vi "Host Approach Retraction2(1)2.vi"() -> ()   [LabVIEW 2012]
uses:
  <vilib>/rvi/interface/nirviOpenFPGA/nirviOpenFPGA.xnode
  <vilib>/rvi/interface/nirviReadWriteControl/nirviReadWriteControl.xnode
  <vilib>/rvi/interface/nirviCloseFPGA/nirviCloseFPGA.xnode
  <vilib>/FPGAPlugInAG/Dynamic/niLvFpga_Close_Dynamic.vi
  <vilib>/rvi/interface/Simulation/niFpgaSimulationCallBeginRW.vi
  <vilib>/rvi/errors/niLvFpgaAdjustHostInterfaceError.vi
  <vilib>/rvi/interface/nirviMethod/nirviMethod.xnode
  <vilib>/FPGAPlugInAG/Dynamic/niLvFpga_Run_Dynamic.vi
  <vilib>/FPGAPlugInAG/PCI-7831R/niLvFpga_Open_PCI-7831R.vi
  <vilib>/rvi/interface/common/dynamic/niFpgaDynamicAddResources.vi
  <vilib>/Utility/error.llb/Error Cluster From Error Code.vi
  <vilib>/rvi/errors/niLvFpgaMergeErrorWithErrorCode.vi
  <vilib>/FPGAPlugInAG/Dynamic/niLvFpga_StartFifo_Dynamic.vi
  <vilib>/FPGAPlugInAG/Dynamic/niLvFpga_StopFifo_Dynamic.vi
  <vilib>/FPGAPlugInAG/Dynamic/niLvFpga_ReadFifo_Dynamic.vi
  SB130-XPS/Documents/FPGA-project-apporach-retraction/FPGA Bitfiles/Apporach-Retract_FPGATarget2_FPGATargetApproa_hZApBjrwAY4.lvbitx
  FPGA Target Approach Retraction2(1).vi
  NiFpgaLv.dll
panel:
  out "H/V  10":i16[](graph)
  out "Tuning Fork Signal":i16[](graph)
  out "Array":i64[](array[numeric])
  in  "Number of Elements":u16
  out "Counter Indicator":i32(graph)
  out "Z Indicator":dbl(graph)
  out "FPGA Output Voltage":dbl(graph)
  in  "MCL Counter":i64
  in  "MCL Divisions":i32
  out "MCL Range Indicator":bool
  out "Host Counter Indicator":i64
  out "Digital Steps per Region":i32
  out "Host Counter Output":i32
  in  "Z Position MCL Fine":i32
  out "Host Z Position Indicator":i32
  out "Z Position Range Indicator":bool
  out "Z Fine Steps per Region":dbl
  out "Host Z Output":fxp<+/-,40,30>
  in  "Manual Approach Start":bool
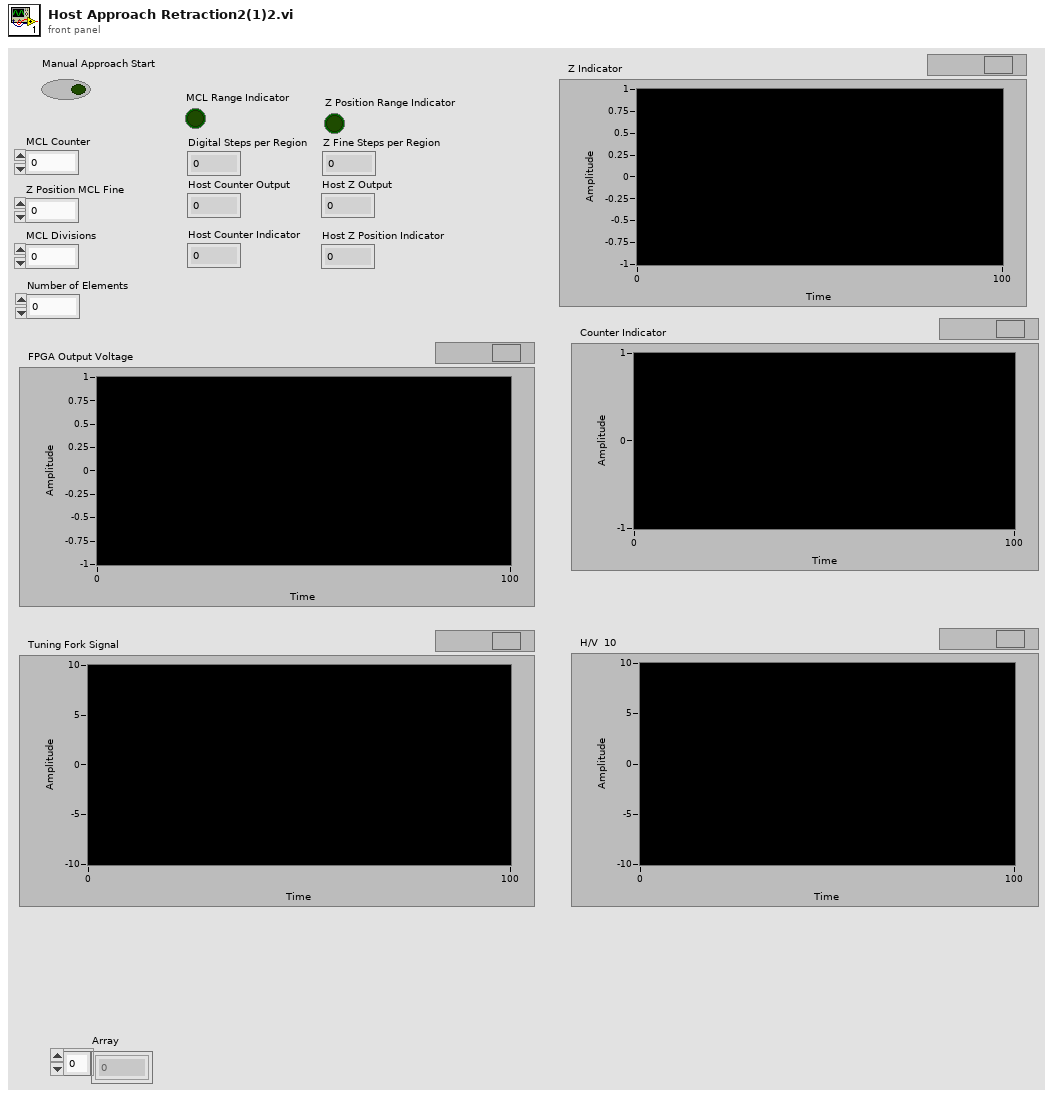
[diagram p1: front panel]
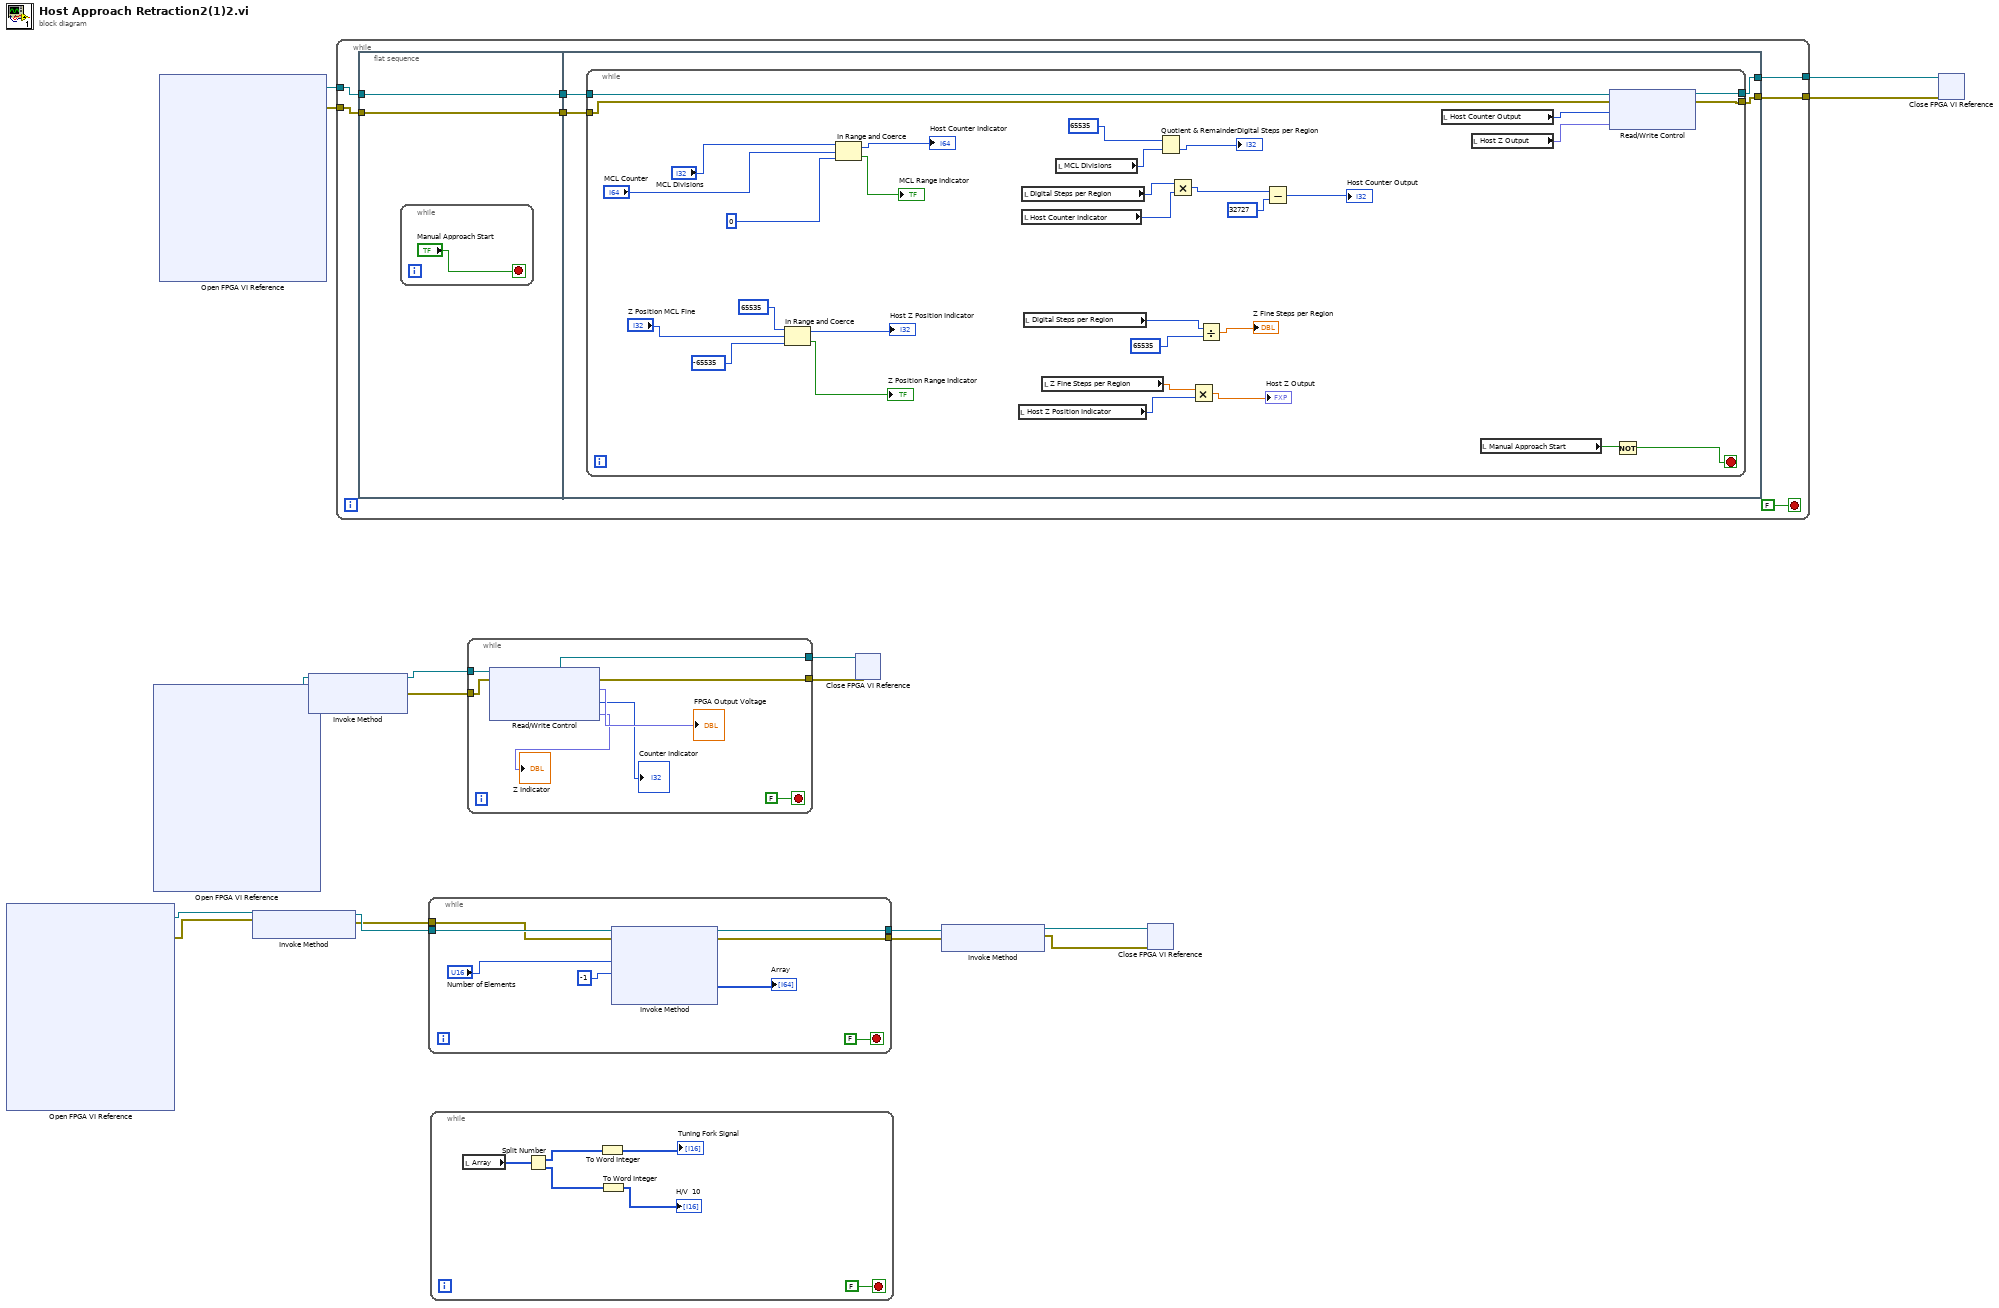
[diagram p0: block diagram]
diagram:
  n1 = xnode "Open FPGA VI Reference"() -> ("FPGA VI Reference Out"=w8:refnum<k20>, "error out"=w7:errorcluster)  [unwired: 2 in]
  n2 = xnode "Open FPGA VI Reference"() -> ("FPGA VI Reference Out"=w10:refnum<k20>, "error out"=w9:errorcluster)  [unwired: 2 in]
  n3 = xnode "Open FPGA VI Reference"() -> ("FPGA VI Reference Out"=w16:refnum<k20>, "error out"=w15:errorcluster)  [unwired: 2 in]
  n4 = xnode "Invoke Method"("FPGA VI Reference In"=w8, "error in"=w7) -> ("FPGA VI Reference Out"=w6:refnum<k20>, "error out"=w5:errorcluster)
  n5 = xnode "Invoke Method"("FPGA VI Reference In"=w10, "error in"=w9) -> ("FPGA VI Reference Out"=w12:refnum<k20>, "error out"=w11:errorcluster)  [unwired: 1 in]
  n6 = while {
    tunnel: [w24] -> w18
    tunnel: [w23] -> w17
    tunnel: w16 -> [w21]
    tunnel: w15 -> [w19]
    stop <- FALSE stop-if-true
    n7 = flat-sequence {
      tunnel: [w27] -> w22
      tunnel: w21 -> [w27]
      tunnel: [w26] -> w20
      tunnel: w19 -> [w26]
      tunnel: [w30] -> w24
      tunnel: [w29] -> w23
      tunnel: w22 -> [w32]
      tunnel: w20 -> [w31]
      frame #0 {
        n8 = while {
          stop <- "Manual Approach Start" stop-if-true
        }
      }
      frame #1 {
        n9 = while {
          tunnel: w32 -> [w64]
          tunnel: w31 -> [w63]
          tunnel: [w62] -> w30
          tunnel: [w61] -> w29
          stop <- w59 stop-if-true
          n10 = In Range and Coerce(upper limit=65535, x="Z Position MCL Fine", lower limit=-65535) -> (coerced(x)=→"Host Z Position Indicator":i32, In Range?=→"Z Position Range Indicator":bool)
          n11 = In Range and Coerce(upper limit="MCL Divisions", x="MCL Counter", lower limit=0) -> (coerced(x)=→"Host Counter Indicator":i64, In Range?=→"MCL Range Indicator":bool)
          n12 = local read "Host Z Position Indicator"() -> (w35:i32)
          n13 = local read "Digital Steps per Region"() -> (w48:i32)
          n14 = local read "Host Counter Indicator"() -> (w47:i64)
          n15 = local read "Digital Steps per Region"() -> (w39:i32)
          n16 = local read "Z Fine Steps per Region"() -> (w36:dbl)
          n17 = local read "MCL Divisions"() -> (w52:i32)
          n18 = Quotient & Remainder(x=65535, y=w52) -> (floor(x/y)=→"Digital Steps per Region":i32)  [unwired: 1 out]
          n19 = Multiply(x=w48, y=w47) -> (x*y=w49:i64)
          n20 = Multiply(x=w36, y=w35) -> (x*y=→"Host Z Output":dbl)
          n21 = Divide(x=w39, y=65535) -> (x/y=→"Z Fine Steps per Region":dbl)
          n22 = Subtract(x=w49, y=32727) -> (x-y=→"Host Counter Output":i64)
          n23 = local read "Host Counter Output"() -> (w45:i32)
          n24 = local read "Host Z Output"() -> (w33:fxp<+/-,40,30>)
          n25 = local read "Manual Approach Start"() -> (w60:bool)
          n26 = xnode "Read/Write Control"("FPGA VI Reference In"=w64, "error in"=w63, "Counter Output"=w45, "Z Fine Output"=w33) -> ("FPGA VI Reference Out"=w62:refnum<k20>, "error out"=w61:errorcluster)
          n27 = Not(x=w60) -> (.not. x?=w59:bool)
        }
      }
    }
  }
  n28 = while {
    tunnel: w6 -> [w72]
    tunnel: w5 -> [w71]
    tunnel: [w70] -> w4
    tunnel: [w69] -> w3
    stop <- FALSE stop-if-true
    n29 = xnode "Invoke Method"("FPGA VI Reference In"=w72, "error in"=w71, "Number of Elements"="Number of Elements", "Timeout (ms)"=-1) -> ("FPGA VI Reference Out"=w70:refnum<k20>, "error out"=w69:errorcluster, "Data"=→"Array":i16[])  [unwired: 1 out]
  }
  n30 = while {
    stop <- FALSE stop-if-true
    n31 = local read "Array"() -> (w78:i64[])
    n32 = Split Number(x=w78) -> (hi(x)=w77:u32[], lo(x)=w76:u32[])
    n33 = To Word Integer(number=w77) -> (16bit integer=→"Tuning Fork Signal":i16[])
    n34 = To Word Integer(number=w76) -> (16bit integer=→"H/V  10":i16[])
  }
  n35 = while {
    tunnel: w12 -> [w85]
    tunnel: w11 -> [w84]
    tunnel: [w83] -> w14
    tunnel: [w82] -> w13
    stop <- FALSE stop-if-true
    n36 = xnode "Read/Write Control"("FPGA VI Reference In"=w85, "error in"=w84) -> ("FPGA VI Reference Out"=w83:refnum<k20>, "error out"=w82:errorcluster, "FPGA Output Voltage"=→"FPGA Output Voltage":fxp<+/-,64,32>, "Counter Indicator"=→"Counter Indicator":i32, "Z Fine Indicator"=→"Z Indicator":fxp<+/-,40,30>)
  }
  n37 = xnode "Close FPGA VI Reference"("FPGA VI Reference In"=w14, "error in"=w13) -> ()  [unwired: 1 out]
  n38 = xnode "Invoke Method"("FPGA VI Reference In"=w4, "error in"=w3) -> ("FPGA VI Reference Out"=w2:refnum<k20>, "error out"=w1:errorcluster)
  n39 = xnode "Close FPGA VI Reference"("FPGA VI Reference In"=w2, "error in"=w1) -> ()  [unwired: 1 out]
  n40 = xnode "Close FPGA VI Reference"("FPGA VI Reference In"=w18, "error in"=w17) -> ()  [unwired: 1 out]
